vi "Read Properties.vi"(8 "error in (no error)":errorcluster, 11 "PropertyNode in":refnum<class "PropertyNode.lvclass">) -> (0 "error out":errorcluster, 2 "Properties":map{string, string}(c390), 3 "PropertyNode out":refnum<class "PropertyNode.lvclass">)   [LabVIEW 2025, in "PropertyNode.lvclass"]
uses:
  PropertyNode.lvclass
  PropertyNode.lvclass/PropertyNode.ctl
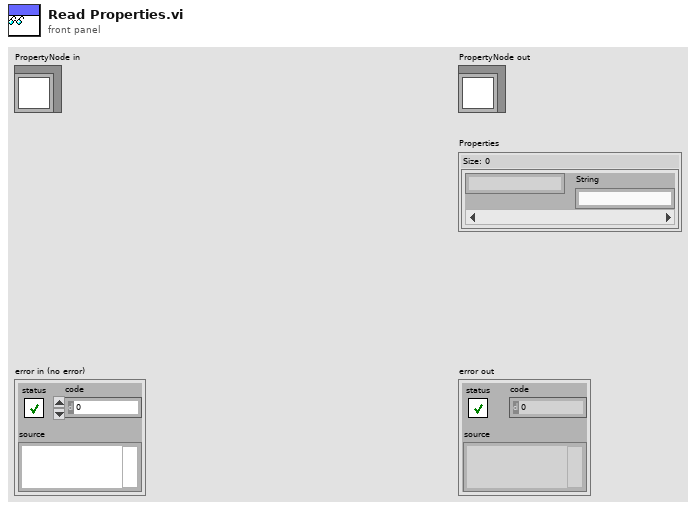
[diagram p1: front panel]
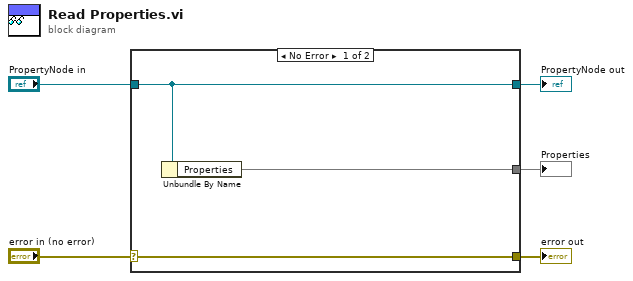
[diagram p0: block diagram]
diagram:
  n1 = case shown="No Error" "error in (no error)" {
    selector: "error in (no error)" -> [w8 w9]
    tunnel: [w8 w9] -> w4
    tunnel: [w7 w10] -> w2
    tunnel: "PropertyNode in" -> [w7 w10]
    tunnel: [w6 _] -> w1
    frame No Error {
      n2 = Unbundle By Name(w7) -> ("Properties"=w6:map{string, string})
    }
    frame Error {
    }
  }
  "error out" <- w4
  "PropertyNode out" <- w2
  "Properties" <- w1
